vi "Configure Brightness of Display.vi"(8 "error in (no error)":errorcluster, 10 "Brightness (0: 100%)":u16(ring) items=["100%", "75%", "50%", "25%", "Display Off", "Display and Indicators Off"], 11 "VISA resource name":refnum<visa-resource-name>) -> (0 "error out":errorcluster, 3 "VISA resource name out":refnum<visa-resource-name>)   [LabVIEW 2017, in "Keithley 2450.lvlib"]
doc: "Sets the brightness of the front-panel display and buttons."
uses:
  Keithley 2450.lvlib
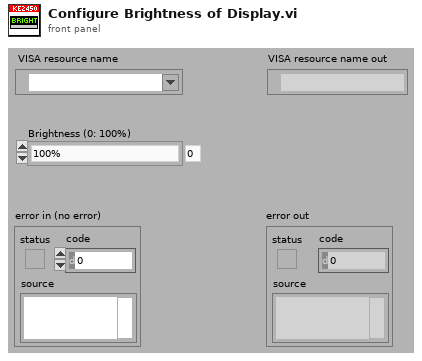
[diagram p1: front panel]
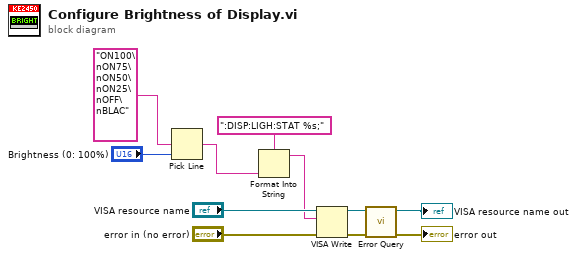
[diagram p0: block diagram]
diagram:
  n1 = Pick Line(multi-line string="ON100\nON75\nON50\nON25\nOFF\nBLAC", line index="Brightness (0: 100%)") -> (output string=w1:string)  [unwired: 1 in]
  n2 = Format Into String(format string=":DISP:LIGH:STAT %s;", w1) -> (resulting string=w4:string)  [unwired: 2 in, 1 out]
  n3 = VISA Write(VISA resource name="VISA resource name", write buffer=w4, error in (no error)="error in (no error)") -> (VISA resource name out=w9:refnum<visa-resource-name>, error out=w6:errorcluster)  [unwired: 1 out]
  n4 = call "Error Query.vi"("error in (no error)"=w6, "VISA resource name"=w9) -> ("error out"=→"error out":errorcluster, "VISA resource name out"=→"VISA resource name out":refnum<visa-resource-name>)  [unwired: 8 out]
